vi "EnterMedidaB.vi"() -> (0 "Frecuencia (seg)":dbl format="%#.1g", 1 "Tiempo de medida (min)":dbl, 3 "Cancelled?":bool)   [LabVIEW 2013]
doc: "Use this template to create a dialog box. This template polls the state of the buttons on the front panel and does not use events. Use the Dialog Using Events template (not available in Base package) to create a dialog box with event handling."
panel:
  in  "Muestreo(s)":dbl=10.0 format="%#.1g"
  in  "Tiempo de medida (min)":dbl=10.0 format="%#.1g"
  in  "Cancel":bool
  in  "OK":bool
  # "Tiempo de medida y \nfrecuencia de toma de datos:"
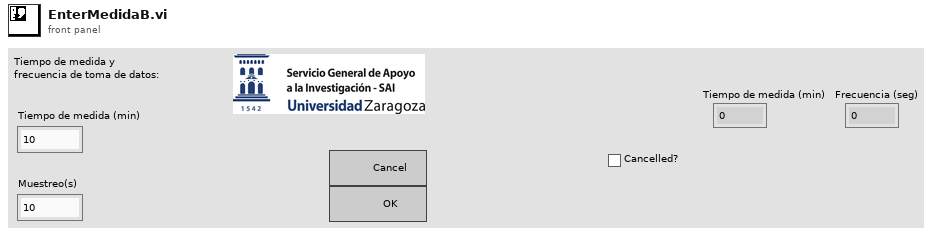
[diagram p1: front panel]
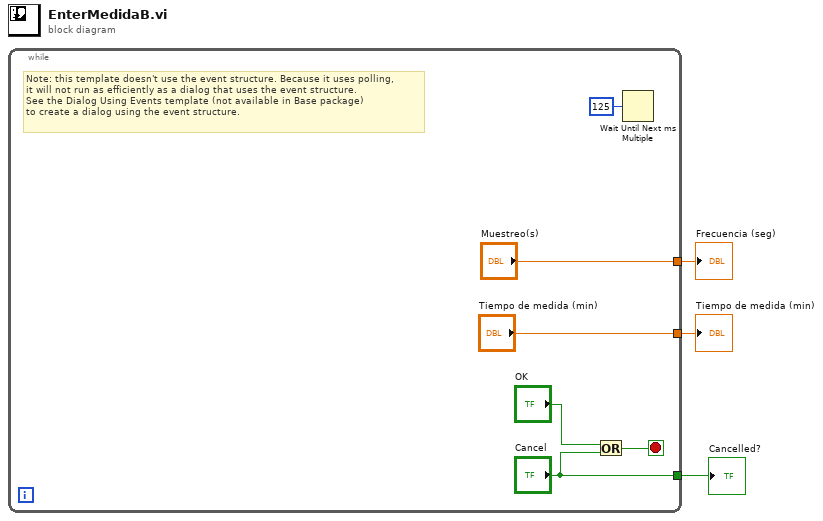
[diagram p0: block diagram]
diagram:
  n1 = while {
    tunnel: ["Cancel"] -> w3
    tunnel: ["Tiempo de medida (min)"] -> w2
    tunnel: ["Muestreo(s)"] -> w1
    stop <- w8 stop-if-true
    # "Note: this template doesn't use the event structure. Because it uses polling, \nit will not run as efficiently as a dialog that uses the event structure.\nSee the Dialog Using Events template (not available in Base package) \nto create a dialog using the event structure."
    n2 = Or(x="OK", y="Cancel") -> (x .or. y?=w8:bool)
    n3 = Wait Until Next ms Multiple(millisecond multiple=u32 125) -> ()  [unwired: 1 out]
  }
  "Cancelled?" <- w3
  "Tiempo de medida (min)" <- w2
  "Frecuencia (seg)" <- w1
